vi "Register Multiple Channel Configs.vi"(0 "Sift Client in":refnum<class "Sift Client.lvclass">, 1 "Channel Configs":T1[](array[typedef]), 2 "Flow Name":string="default_flow_name", 3 "Asset Name":string, 4 "Submit Ingestion Config":bool, 5 "error in (no error)":errorcluster) -> (14 "Sift Client out":refnum<class "Sift Client.lvclass">, 15 "Ingestion Config ID":string, 19 "error out":errorcluster)   [LabVIEW 2024, in "Sift Client.lvlib" / "Sift Client.lvclass"]
uses:
  Sift Client.lvclass
  Private/Typedefs/Ingestion Config/Channel Config.ctl
  Types/Data Type.ctl
  Types/Bit Field.ctl
  Types/Enum.ctl
  Sift Client.lvlib
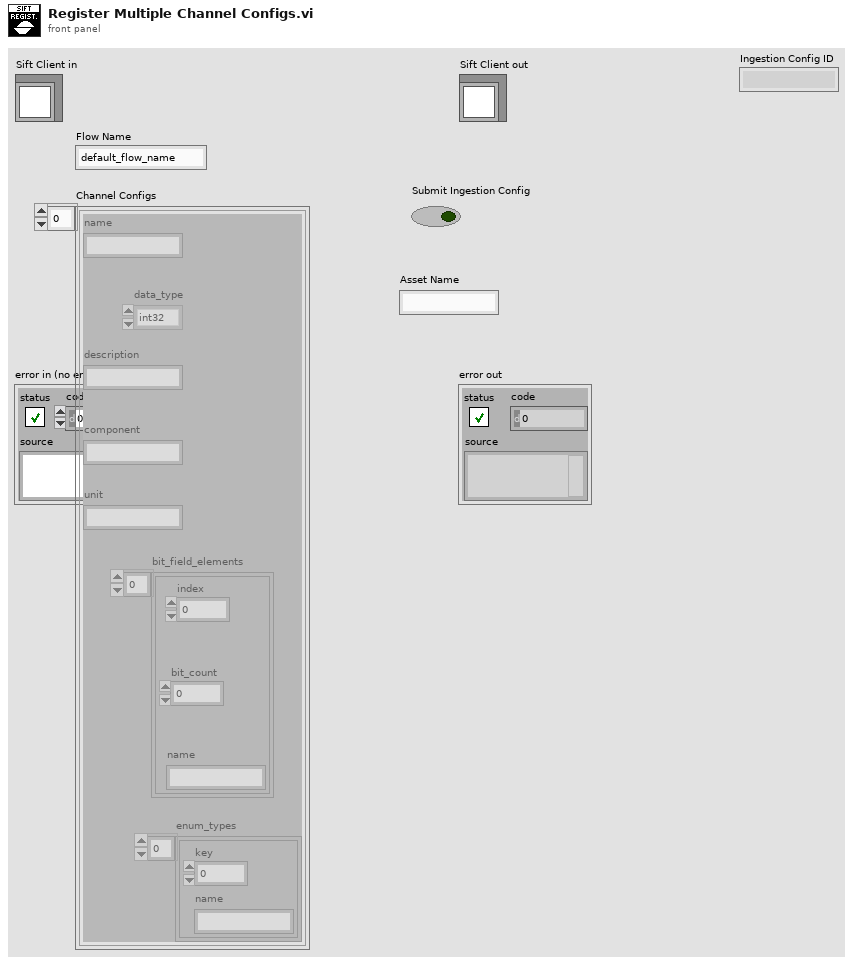
[diagram p1: front panel]
types:
  T1 = typedef "Sift Client.lvlib/Channel Config.ctl" = cluster{"name":string, "data_type":T2, "description":string, "component":string, "unit":string, "bit_field_elements":T3[], "enum_types":T4[]}
  T2 = typedef "Sift Client.lvlib/Data Type.ctl" = enum8{"double", "float", "uint64", "int64", "uint32", "int32", "bool", "enum", "string"}
  T3 = typedef "Bit Field.ctl" = cluster{"index":u32, "bit_count":u32, "name":string}
  T4 = typedef "Sift Client.lvlib/Enum.ctl" = cluster{"key":u32, "name":string}
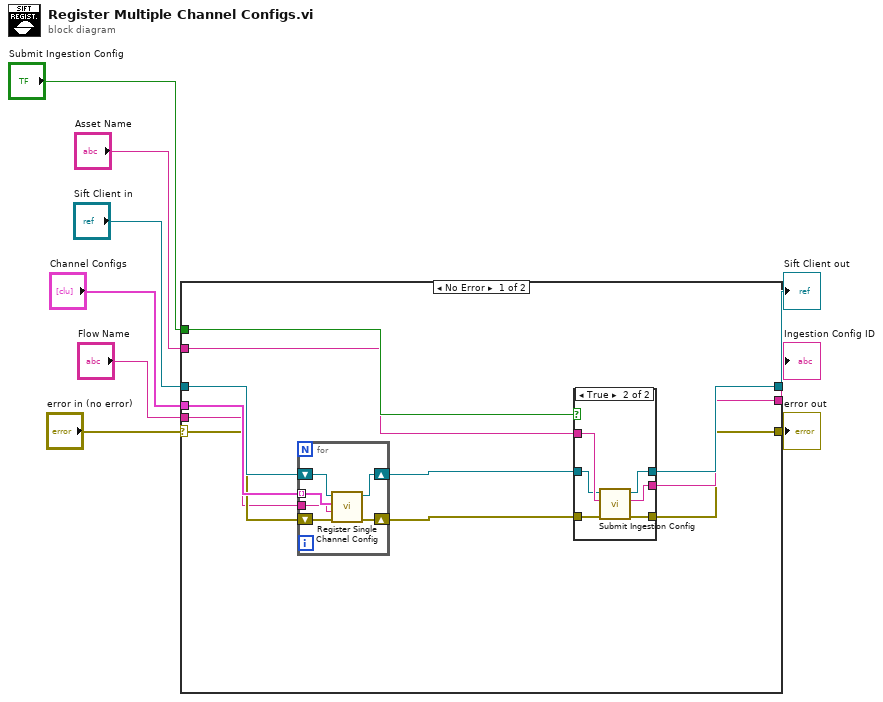
[diagram p0: block diagram]
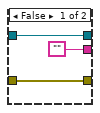
[diagram p2: hidden frame]
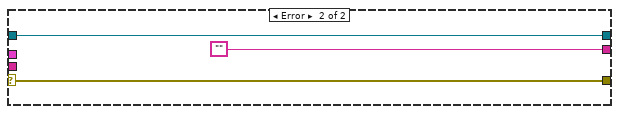
[diagram p3: hidden frame]
diagram:
  n1 = case shown="No Error" "error in (no error)" {
    selector: "error in (no error)" -> [w18 w38]
    tunnel: [w11 w38] -> w8
    tunnel: [w13 w37] -> w6
    tunnel: "Sift Client in" -> [w19 w37]
    tunnel: "Channel Configs" -> [w20 _]
    tunnel: "Submit Ingestion Config" -> [w17 _]
    tunnel: "Asset Name" -> [w15 _]
    tunnel: [w12 ""] -> w2
    tunnel: "Flow Name" -> [w10 _]
    frame No Error {
      n2 = for {
        tunnel: w20 -> [w35] mode=indexing
        tunnel: w10 -> [w30]
        shift-right: [w31] -> w16
        shift-left: w18 -> [w32]
        shift-right: [w33] -> w14
        shift-left: w19 -> [w34]
        n3 = call-dynamic "Register Single Channel Config.vi"("error in (no error)"=w32, "Flow Name"=w30, "Channel Config"=w35, "Sift Client in"=w34) -> ("error out"=w31:errorcluster, "Sift Client out"=w33:refnum<class "Sift Client.lvclass">)  [unwired: 6 in]
      }
      n4 = case shown="True" w17 {
        tunnel: w16 -> [w21 w29]
        tunnel: w15 -> [_ w28]
        tunnel: w14 -> [w23 w27]
        tunnel: [w23 w26] -> w13
        tunnel: ["" w25] -> w12
        tunnel: [w21 w24] -> w11
        frame False {
        }
        frame True {
          n5 = call-dynamic "Submit Ingestion Config.vi"("error in (no error)"=w29, "Asset Name"=w28, "Sift Client in"=w27) -> ("error out"=w24:errorcluster, "Ingestion Config ID"=w25:string, "Sift Client out"=w26:refnum<class "Sift Client.lvclass">)  [unwired: 6 in]
        }
      }
    }
    frame Error {
    }
  }
  "error out" <- w8
  "Sift Client out" <- w6
  "Ingestion Config ID" <- w2
